vi "Create_individual_plot_Titles.vi"(7 "Swop Series and Plots":bool) -> (0 "2D Plot Titles":string[](array[string]), 1 "1D Plot Titles":string[](array[string]), 2 "Desired Legends":string[][](array[string]), 3 "Plot Legends Auto":string[](array[string]), 4 "Dont show axis label":bool)   [LabVIEW 2022 SP3]
uses:
  Choose_Title.ctl
  Anemometry/Anemometry Sub Vis/Data_plotting_vis/Results_plotter_Global.vi
panel:
  in  "Cluster":T1
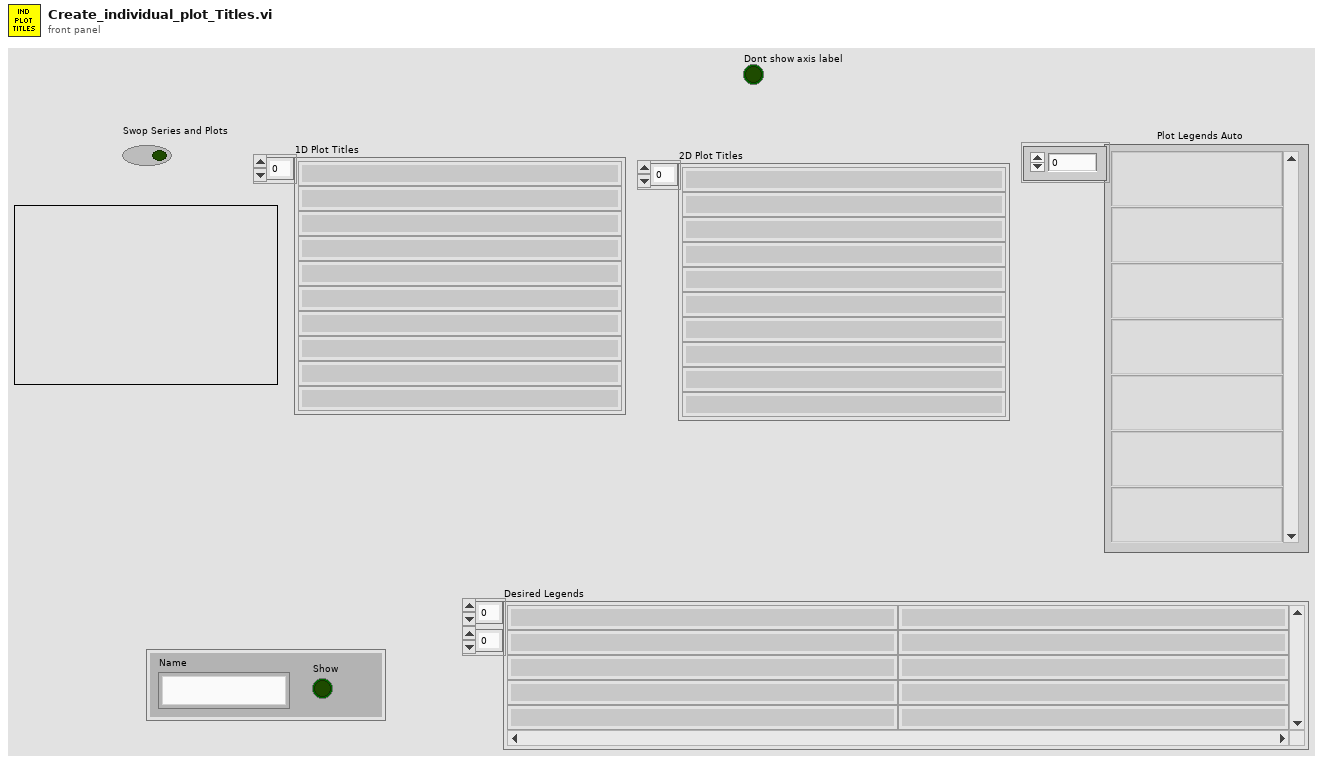
[diagram p1: front panel]
types:
  T1 = typedef "Choose_Title.ctl" = cluster{"Name":string, "Show":bool}
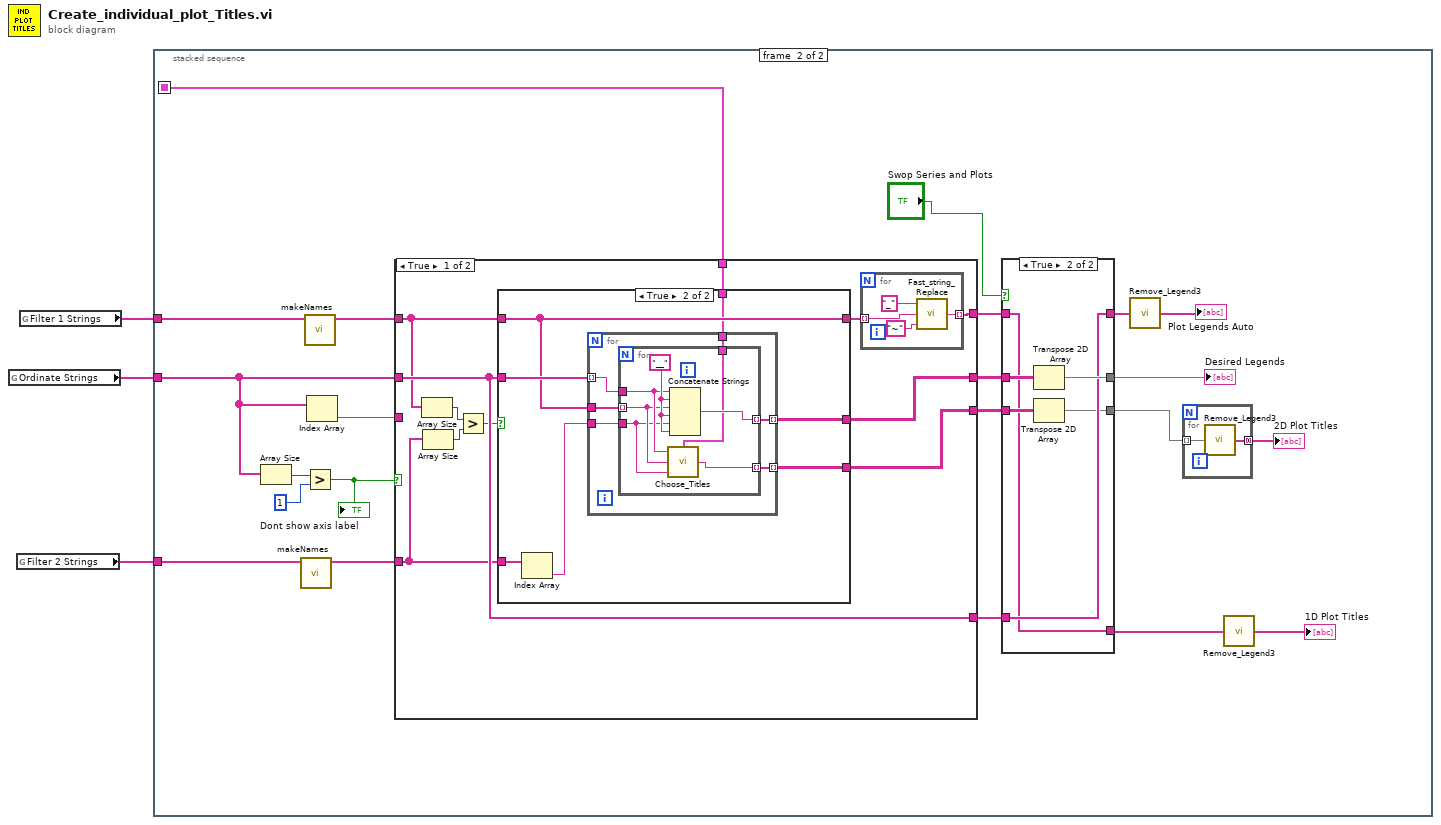
[diagram p0: block diagram]
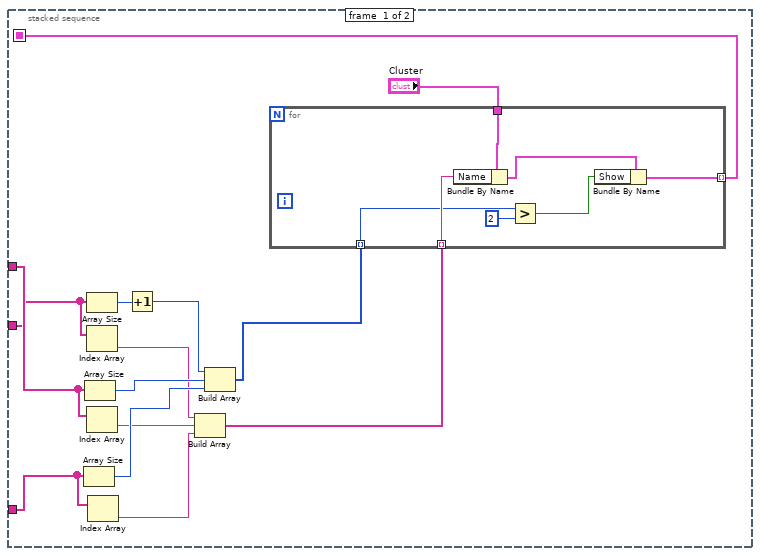
[diagram p2: hidden frame]
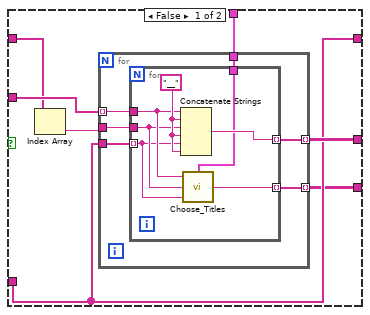
[diagram p4: hidden frame]
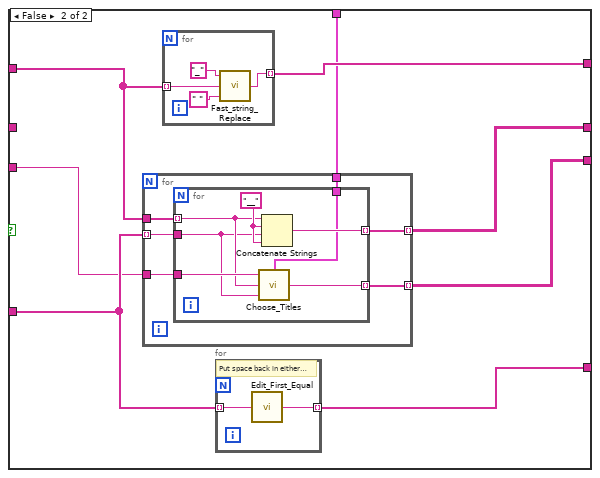
[diagram p5: hidden frame]
diagram:
  n1 = global read "Results_plotter_Global.vi" "Ordinate Strings"() -> (w1:string[])
  n2 = global read "Results_plotter_Global.vi" "Filter 2 Strings"() -> (w2:string[])
  n3 = global read "Results_plotter_Global.vi" "Filter 1 Strings"() -> (w3:string[])
  n4 = stacked-sequence {
    seq-local: [w5 _] -> [_ w30]
    tunnel: w3 -> [w8 w33]
    tunnel: w2 -> [w7 w31]
    tunnel: w1 -> [w6 w32]
    frame #0 {
      n5 = Array Size(array=w7) -> (size(s)=w14:i32)
      n6 = Array Size(array=w8) -> (size(s)=w13:i32)
      n7 = Array Size(array=w6) -> (size(s)=w12:i32)
      n8 = Index Array(array=w6) -> (element=w9:string)  [unwired: 1 in]
      n9 = Index Array(array=w8) -> (element=w10:string)  [unwired: 1 in]
      n10 = Index Array(array=w7) -> (element=w11:string)  [unwired: 1 in]
      n11 = Increment(x=w12) -> (x+1=w17:i32)
      n12 = Build Array(w9, w10, w11) -> (w15:string[])
      n13 = Build Array(w17, w13, w14) -> (w16:i32[])
      n14 = for {
        tunnel: w15 -> [w24] mode=indexing
        tunnel: w16 -> [w23] mode=indexing
        tunnel: [w20] -> w5 mode=indexing
        tunnel: "Cluster" -> [w18]
        n15 = Bundle By Name(cluster=w18, "Name"=w24) -> (w21:T1)
        n16 = Greater?(x=w23, y=2) -> (0:w19:bool)
        n17 = Bundle By Name(cluster=w21, "Show"=w19) -> (w20:T1)
      }
    }
    frame #1 {
      n18 = Array Size(array=w32) -> (size(s)=w34:i32)
      n19 = call "makeNames.vi"("Strings"=w31) -> ("Names"=w37:string[])  [unwired: 10 in]
      n20 = call "makeNames.vi"("Strings"=w33) -> ("Names"=w38:string[])  [unwired: 10 in]
      n21 = Greater?(x=w34, y=1) -> (0:w36:bool)
      "Dont show axis label" <- w36
      n22 = Index Array(array=w32) -> (element=w46:string)  [unwired: 1 in]
      n23 = case shown="True" w36 {
        tunnel: w38 -> [w64 w117]
        tunnel: w37 -> [w65 w118]
        tunnel: [w61 w121] -> w39
        tunnel: [w68 w120] -> w40
        tunnel: [w69 w119] -> w44
        tunnel: w32 -> [w68 _]
        tunnel: w30 -> [w60 w115]
        tunnel: [w59 w114] -> w45
        tunnel: w46 -> [_ w116]
        frame True {
          n24 = Array Size(array=w64) -> (size(s)=w67:i32)
          n25 = Array Size(array=w65) -> (size(s)=w66:i32)
          n26 = Greater?(x=w67, y=w66) -> (0:w63:bool)
          n27 = case shown="True" w63 {
            tunnel: [w79 w100] -> w69
            tunnel: w68 -> [w78 w99]
            tunnel: w65 -> [w76 w98]
            tunnel: w64 -> [w77 w96]
            tunnel: [w76 w96] -> w62
            tunnel: w60 -> [w75 w94]
            tunnel: [w74 w95] -> w59
            frame False {
              n28 = Index Array(array=w77) -> (element=w80:string)  [unwired: 1 in]
              n29 = for {
                tunnel: w80 -> [w86]
                tunnel: w76 -> [w85]
                tunnel: [w84] -> w79 mode=indexing
                tunnel: w78 -> [w83] mode=indexing
                tunnel: w75 -> [w82]
                tunnel: [w81] -> w74 mode=indexing
                n30 = for {
                  tunnel: w86 -> [w90]
                  tunnel: w85 -> [w89] mode=indexing
                  tunnel: [w93] -> w84 mode=indexing
                  tunnel: w83 -> [w91]
                  tunnel: w82 -> [w88]
                  tunnel: [w87] -> w81 mode=indexing
                  w92 = "__" ("string")
                  n31 = Concatenate Strings(w91, w92, w90, w92, w89, w92) -> (w93:string)
                  n32 = call "Choose_Titles.vi"("Titles to Show"=w88, "String 3"=w89, "String 2"=w90, "String1"=w91) -> ("Title"=w87:string)
                }
              }
            }
            frame True {
              n33 = Index Array(array=w98) -> (element=w97:string)  [unwired: 1 in]
              n34 = for {
                tunnel: w96 -> [w106]
                tunnel: w97 -> [w105]
                tunnel: [w104] -> w100 mode=indexing
                tunnel: w99 -> [w103] mode=indexing
                tunnel: [w102] -> w95 mode=indexing
                tunnel: w94 -> [w101]
                n35 = for {
                  tunnel: w106 -> [w110] mode=indexing
                  tunnel: w105 -> [w109]
                  tunnel: [w113] -> w104 mode=indexing
                  tunnel: w103 -> [w111]
                  tunnel: [w108] -> w102 mode=indexing
                  tunnel: w101 -> [w107]
                  w112 = "__" ("string")
                  n36 = call "Choose_Titles.vi"("Titles to Show"=w107, "String 3"=w109, "String 2"=w110, "String1"=w111) -> ("Title"=w108:string)
                  n37 = Concatenate Strings(w111, w112, w110, w112, w109, w112) -> (w113:string)
                }
              }
            }
          }
          n38 = for {
            tunnel: w62 -> [w72] mode=indexing
            tunnel: [w71] -> w61 mode=indexing
            n39 = call "Fast_string_Replace.vi"("Replace match with:"="~", "Input String"=w72, "matchThis"="_" ("regular expression")) -> ("Output String"=w71:string)  [unwired: 1 in, 1 out]
          }
        }
        frame False {
          n40 = for {
            tunnel: w117 -> [w133]
            tunnel: w118 -> [w132] mode=indexing
            tunnel: [w131] -> w119 mode=indexing
            tunnel: w116 -> [w130]
            tunnel: w115 -> [w129]
            tunnel: [w128] -> w114 mode=indexing
            n41 = for {
              tunnel: w133 -> [w137] mode=indexing
              tunnel: w132 -> [w136]
              tunnel: [w139] -> w131 mode=indexing
              tunnel: w130 -> [w138]
              tunnel: w129 -> [w135]
              tunnel: [w134] -> w128 mode=indexing
              w140 = "__" ("string")
              n42 = call "Choose_Titles.vi"("Titles to Show"=w135, "String 3"=w136, "String 2"=w137, "String1"=w138) -> ("Title"=w134:string)
              n43 = Concatenate Strings(w137, w140, w136, w140) -> (w139:string)
            }
          }
          n44 = for {
            tunnel: w117 -> [w123] mode=indexing
            tunnel: [w122] -> w121 mode=indexing
            n45 = call "Fast_string_Replace.vi"("Replace match with:"=" ", "Input String"=w123, "matchThis"="_" ("regular expression")) -> ("Output String"=w122:string)  [unwired: 1 in, 1 out]
          }
          n46 = for {
            tunnel: w118 -> [w127] mode=indexing
            tunnel: [w126] -> w120 mode=indexing
            # "Put space back in either side of the = sign"
            n47 = call "Edit_First_Equal.vi"("String in"=w127) -> ("String out"=w126:string)
          }
        }
      }
      n48 = case shown="True" "Swop Series and Plots" {
        tunnel: w44 -> [w52 w58]
        tunnel: [w52 w57] -> w43
        tunnel: [w51 w56] -> w41
        tunnel: w39 -> [w51 w53]
        tunnel: w40 -> [w49 w56]
        tunnel: [w50 w54] -> w28
        tunnel: w45 -> [w50 w55]
        tunnel: [w49 w53] -> w27
        frame False {
        }
        frame True {
          n49 = Transpose 2D Array(2D array=w58) -> (transposed array=w57:string[][])
          n50 = Transpose 2D Array(2D array=w55) -> (transposed array=w54:string[][])
        }
      }
      "Desired Legends" <- w43
      n51 = call "Remove_Legend3.vi"("Ordinate Strings"=w41) -> ("Array"=→"Plot Legends Auto":string[])
      n52 = for {
        tunnel: w28 -> [w48] mode=indexing
        tunnel: [w47] -> w25 mode=concatenating
        n53 = call "Remove_Legend3.vi"("Ordinate Strings"=w48) -> ("Array"=w47:string[])
      }
      "2D Plot Titles" <- w25
      n54 = call "Remove_Legend3.vi"("Ordinate Strings"=w27) -> ("Array"=→"1D Plot Titles":string[])
    }
  }
